vi "VerifyArguments.vi"(8 "error in (no error)":errorcluster, 11 "SecureRunVI in":refnum<class "SecureRunVI.lvclass">) -> (0 "error out":errorcluster, 3 "SecureRunVI out":refnum<class "SecureRunVI.lvclass">)   [LabVIEW 2023, in "SecureRunVI.lvclass"]
doc: "Ensures required arguments are provided to the LabVIEWCLI."
uses:
  SecureRunVI.lvclass
  SecureRunVI.lvclass/SecureRunVI.ctl
  C:/Program Files (x86)/National Instruments/Shared/LabVIEW CLI/Operations/Utilities/OperationErrorType.ctl
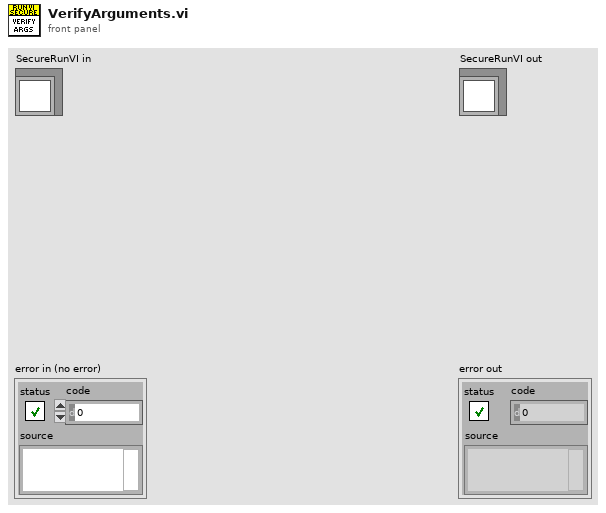
[diagram p1: front panel]
types:
  T1 = typedef "OperationErrorType.ctl" = enum16{"RequiredArgumentMissing", "UnknownArguments", "LoggerSetMultipleTimes", "OperationBrokenError"}
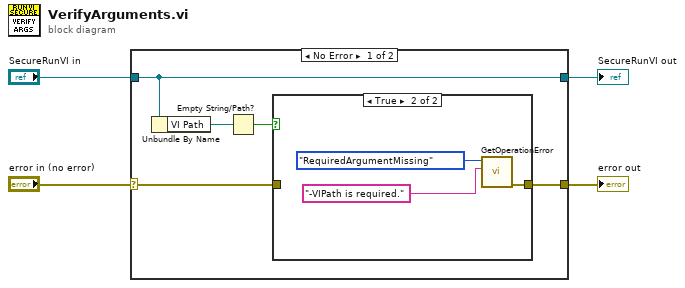
[diagram p0: block diagram]
diagram:
  n1 = case shown="No Error" "error in (no error)" {
    selector: "error in (no error)" -> [w7 w15]
    tunnel: [w6 w15] -> w3
    tunnel: [w5 w14] -> w1
    tunnel: "SecureRunVI in" -> [w5 w14]
    frame No Error {
      n2 = Unbundle By Name(w5) -> ("VI Path"=w9:path)
      n3 = Empty String/Path?(string/path=w9) -> (empty?=w8:bool)
      n4 = case shown="True" w8 {
        tunnel: w7 -> [w10 _]
        tunnel: [w10 w13] -> w6
        frame False {
        }
        frame True {
          n5 = call "GetOperationError.vi"("Additional Information"="-VIPath is required.", "Operation Error Type"=OperationErrorType."RequiredArgumentMissing") -> ("error out"=w13:errorcluster)  [unwired: 9 in]
        }
      }
    }
    frame Error {
    }
  }
  "error out" <- w3
  "SecureRunVI out" <- w1
